vi "Button Notifier Set.vi"   [LabVIEW 2013]
uses:
  <vilib>/Rock Robotics/WPI/Joystick/WPI_JoystickGetSetRefNum.vi
types:
  T1 = typedef "WPI_JoystickDevRef.ctl" = cluster{"Device":T2}
  T2 = typedef "WPI_JoystickDeviceEnum.ctl" = enum16{"USB 1", "USB 2", "USB 3", "USB 4", "Kinect 1", "Kinect 2"}
  T3 = typedef "WPI_JoystickButtonState.ctl" = cluster{"Button 1":bool, "Button 2":bool, "Button 3":bool, "Button 4":bool, "Button 5":bool, "Button 6":bool, "Button 7":bool, "Button 8":bool, "Button 9":bool, "Button 10":bool, "Button 11":bool, "Button 12":bool}
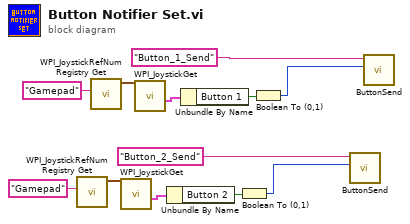
[diagram p0: block diagram]
diagram:
  n1 = call <vilib>:"WPI_JoystickRefNum Registry Get.vi"("refnum name"="Gamepad") -> ("JoystickDevRef"=w9:T1)  [unwired: 9 in, 1 out]
  n2 = call <vilib>:"WPI_JoystickRefNum Registry Get.vi"("refnum name"="Gamepad") -> ("JoystickDevRef"=w3:T1)  [unwired: 9 in, 1 out]
  n3 = call <vilib>:"WPI_JoystickGet.vi"("JoystickDevRef"=w9) -> ("Buttons"=w10:T3)  [unwired: 4 in, 2 out]
  n4 = call <vilib>:"WPI_JoystickGet.vi"("JoystickDevRef"=w3) -> ("Buttons"=w4:T3)  [unwired: 4 in, 2 out]
  n5 = Unbundle By Name(w10) -> ("Button 2"=w11:bool)
  n6 = Unbundle By Name(w4) -> ("Button 1"=w5:bool)
  n7 = Boolean To (0,1)(Boolean=w11) -> (0, 1=w12:i16)
  n8 = Boolean To (0,1)(Boolean=w5) -> (0, 1=w6:i16)
  n9 = call "ButtonSend.vi"("Button Value"=w12, "Notifier Name"="Button_2_Send") -> ()  [unwired: 9 in, 1 out]
  n10 = call "ButtonSend.vi"("Button Value"=w6, "Notifier Name"="Button_1_Send") -> ()  [unwired: 9 in, 1 out]
